vi "setUp.vi"(8 "error in (no error)":errorcluster, 11 "reference in":refnum<class "Disabled Custom Device.lvclass">) -> (0 "error out":errorcluster, 3 "reference out":refnum<class "Disabled Custom Device.lvclass">)   [LabVIEW 2020, in "Disabled Custom Device.lvclass"]
doc: "setUp runs prior to the test method during test execution. Use this method to initialize any object data required by your tests."
uses:
  Disabled Custom Device.lvclass
  C:/Program Files (x86)/National Instruments/LabVIEW 2020/vi.lib/addons/_JKI Toolkits/VI Tester/TestCase.llb/TestCase.lvclass
  Disabled Custom Device.lvclass/Disabled Custom Device.ctl
  <vilib>/addons/_JKI Toolkits/VI Tester/TestCase.llb/TestCase.lvclass
  niveristand-custom-device-testing-tools/VeriStandTestUtilities/VeriStandTestUtilities.lvlib
  Scripting/Ballard MIL-STD-1553 Scripting.lvlib
  C:/dev/git/niveristand-custom-device-testing-tools/VeriStandTestCase/VeriStandTestCase.lvclass
  C:/dev/git/niveristand-ballard-milStd1553-custom-device/Source/Custom Device Support/Tests/System/Disabled Custom Device/Disabled Custom Device.lvclass
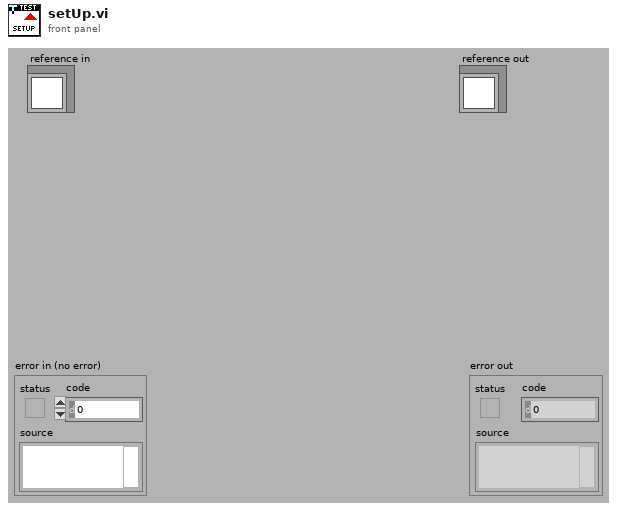
[diagram p1: front panel]
types:
  T1 = typedef "Custom Device API.lvlib/Custom Device Item Ref.ctl" = u64
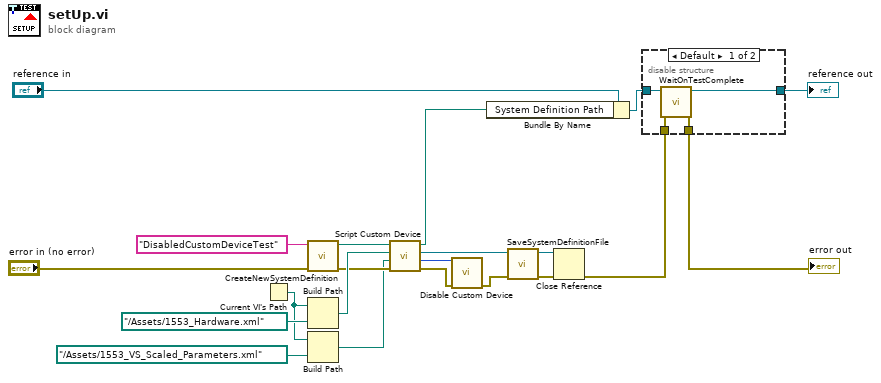
[diagram p0: block diagram]
diagram:
  n1 = Current VI's Path() -> (path=w4:path)
  n2 = call "CreateNewSystemDefinition.vi"("error in"="error in (no error)", "System Definition Name"="DisabledCustomDeviceTest" ("Channel")) -> ("error out"=w10:errorcluster, "System Definition Path"=w9:path)  [unwired: 8 in]
  n3 = Build Path(base path=w4, name or relative path=path "../Assets/1553_Hardware.xml" ("Hardware File Path")) -> (appended path=w14:path)
  n4 = Build Path(base path=w4, name or relative path=path "../Assets/1553_VS_Scaled_Parameters.xml" ("Hardware File Path")) -> (appended path=w5:path)
  n5 = call "Script Custom Device.vi"("error in"=w10, "parameters configuration file path"=w5, "hardware configuration file path"=w14, "system definition path in"=w9) -> ("error out"=w2:errorcluster, "Ballard MIL-STD 1553 custom device out"=w3:T1, "System Definition"=w8:refnum<k24>, "system definition path out"=w15:path)  [unwired: 4 in]
  n6 = call "Disable Custom Device.vi"("error in"=w2, "Ballard MIL-STD 1553 custom device in"=w3) -> ("error out"=w1:errorcluster)  [unwired: 8 in, 1 out]
  n7 = Bundle By Name(cluster="reference in", "System Definition Path"=w15) -> (w17:refnum<class "Disabled Custom Device.lvclass">)
  n8 = call "SaveSystemDefinitionFile.vi"("error in (no error)"=w1, "System Definition Reference in"=w8) -> ("error out"=w7:errorcluster, "System Definition Reference out"=w6:refnum<k24>)  [unwired: 8 in]
  n9 = Close Reference(reference=w6, error in (no error)=w7) -> (error out=w16:errorcluster)
  n10 = disable-structure shown="Default" {
    disable-tunnel: w16 -> [w25 w26]
    disable-tunnel: [w24 w26] -> w21
    disable-tunnel: [w23 w27] -> w19
    disable-tunnel: w17 -> [w22 w27]
    frame condition #0 (active) {
      n11 = call <vilib>:"WaitOnTestComplete.vi"("error in (no error)"=w25, "TestCase in"=w22) -> ("error out"=w24:errorcluster, "TestCase out"=w23:refnum<class "Disabled Custom Device.lvclass">)  [unwired: 8 in]
    }
    frame condition #1 {
    }
  }
  "error out" <- w21
  "reference out" <- w19
